vi "StudentScope - Voltage Range Convert.vi"(0 "Input Voltage Range":u16) -> (1 "V min":i32, 2 "V max":i32)   [LabVIEW 2015]
doc: "This VI converts an input voltage range of enum type to high and low limits sent to the DAQ VIs."
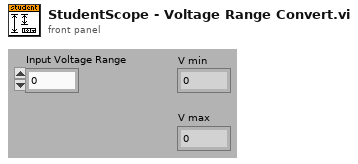
[diagram p1: front panel]
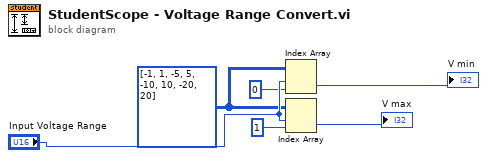
[diagram p0: block diagram]
diagram:
  w1 = i32[][] [[-1, 1], [-5, 5], [-10, 10], [-20, 20]]
  n1 = Index Array(array=w1, index (row)="Input Voltage Range", index (col)=0 ("disabled index (col)")) -> (element=→"V min":i32)
  n2 = Index Array(array=w1, index (row)="Input Voltage Range", index (col)=1 ("disabled index (col)")) -> (element=→"V max":i32)
